vi "Initialize Tecan.vi"(7 "Address":u8, 8 "error IO":errorcluster, 11 "VISA resource name":refnum<visa-resource-name>="COM3") -> (0 "error out":errorcluster, 1 "Status Code":string, 2 "Connected":bool, 3 "VISA resource name Out":refnum<visa-resource-name>)   [LabVIEW 2018]
panel:
  out "Value":dbl
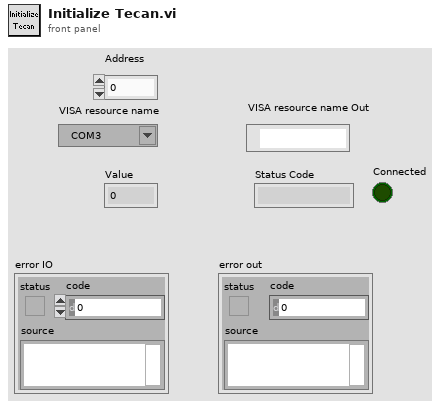
[diagram p1: front panel]
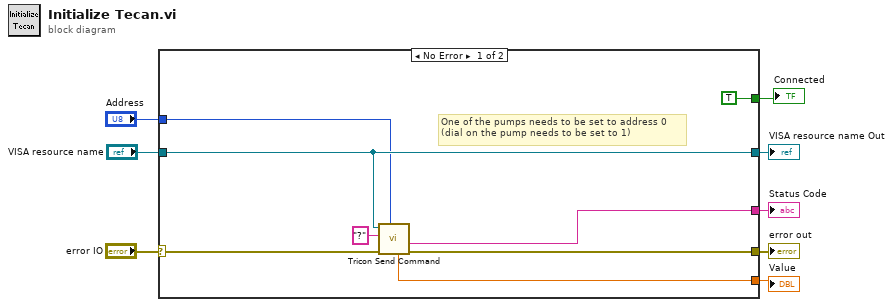
[diagram p0: block diagram]
diagram:
  n1 = case shown="No Error" "error IO" {
    selector: "error IO" -> [w15 w17]
    tunnel: [w14 w17] -> w8
    tunnel: "VISA resource name" -> [w13 _]
    tunnel: [w13 _] -> w5
    tunnel: [w12 _] -> w3
    tunnel: [w11 _] -> w4
    tunnel: [TRUE ("Connected") _] -> w2
    tunnel: "Address" -> [w9 _]
    frame No Error {
      # "One of the pumps needs to be set to address 0\n(dial on the pump needs to be set to 1)"
      n2 = call "Tricon Send Command.vi"("Address"=w9, "error in (no error)"=w15, "Command"="?", "VISA resource name in"=w13) -> ("error out"=w14:errorcluster, "Status Code"=w11:string, "Value"=w12:dbl)  [unwired: 3 in, 2 out]
    }
    frame Error {
    }
  }
  "error out" <- w8
  "VISA resource name Out" <- w5
  "Status Code" <- w4
  "Value" <- w3
  "Connected" <- w2
